vi "Laplace Inverse CDF.vi"(9 "b":dbl=1.0, 10 "a":dbl, 11 "cdf(x)":dbl=0.6) -> (0 "error":i32, 3 "x":dbl=0.2231435513142097)   [LabVIEW 2020, in "NI_Gmath.lvlib"]
doc: "Computes the continuous inverse cumulative distribution function (CDF) of the various distributions. You must manually select the polymorphic instance to use."
uses:
  NI_Gmath.lvlib
  st_error_code.ctl
panel:
  # "Laplace Inverse CDF"
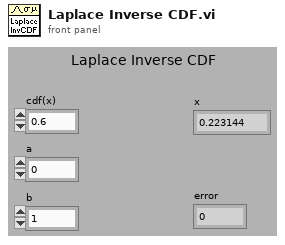
[diagram p1: front panel]
types:
  T1 = typedef "NI_Gmath.lvlib/st_error_code.ctl" = i32
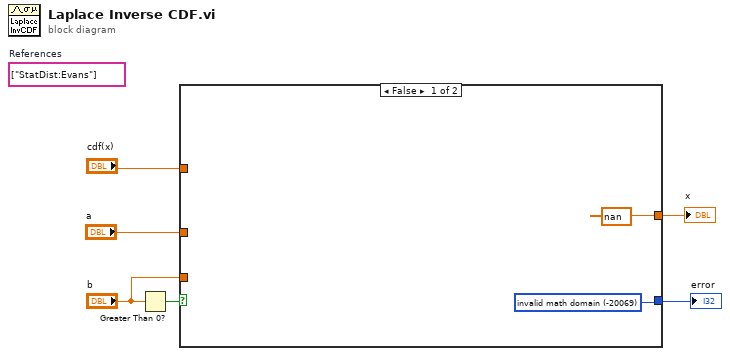
[diagram p0: block diagram]
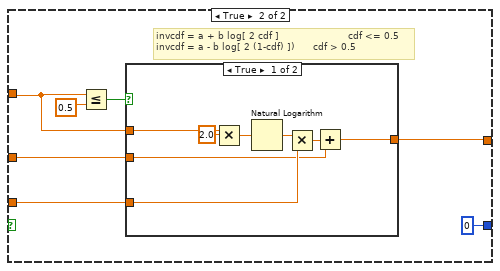
[diagram p2: hidden frame]
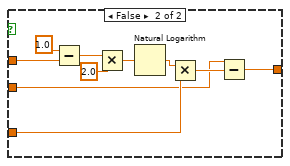
[diagram p3: hidden frame]
diagram:
  (unwired) string[] ["StatDist:Evans"]  # References
  n1 = Greater Than 0?(x="b") -> (x > 0?=w1:bool)
  n2 = case shown="False" w1 {
    tunnel: "b" -> [_ w13]
    tunnel: [w7 0 ("invalid math domain")] -> w2
    tunnel: [nan w12] -> w3
    tunnel: "cdf(x)" -> [_ w11]
    tunnel: "a" -> [_ w9]
    frame False {
      w7 = T1 -20069 items=["invalid math domain"=-20069, "Fourier interpolation size m >= n"=-20070, "empty array"=-20003] ("stat interp error code")
    }
    frame True {
      # "invcdf = a + b log[ 2 cdf ]                       cdf <= 0.5\ninvcdf = a - b log[ 2 (1-cdf) ])      cdf > 0.5"
      n3 = Less Or Equal?(x=w11, y=0.5) -> (x <= y?=w10:bool)
      n4 = case shown="True" w10 {
        tunnel: w13 -> [w22 w32]
        tunnel: [w19 w24] -> w12
        tunnel: w11 -> [w17 w29]
        tunnel: w9 -> [w16 w25]
        frame True {
          n5 = Multiply(x=w17, y=2.0) -> (x*y=w23:dbl)
          n6 = Natural Logarithm(1:w23) -> (0:w21:dbl)
          n7 = Multiply(x=w21, y=w22) -> (x*y=w20:dbl)
          n8 = Add(x=w20, y=w16) -> (x+y=w19:dbl)
        }
        frame False {
          n9 = Subtract(x=1.0 ("y"), y=w29) -> (x-y=w28:dbl)
          n10 = Multiply(x=w28, y=2.0) -> (x*y=w33:dbl)
          n11 = Natural Logarithm(1:w33) -> (0:w31:dbl)
          n12 = Multiply(x=w31, y=w32) -> (x*y=w26:dbl)
          n13 = Subtract(x=w25, y=w26) -> (x-y=w24:dbl)
        }
      }
    }
  }
  "x" <- w3
  "error" <- w2
